vi "subItemInfoToLinkerInfo.vi"(11 "Item info[]":T1[](array[typedef])) -> (3 "Linker.Read Info From File":T3(array[cluster]))   [LabVIEW 2020, in "Tests.DependencyInspection.lvlib"]
uses:
  Tests.DependencyInspection.lvlib
  <vilib>/Utility/lvfile.llb/LVFileType.ctl
  <vilib>/Utility/lvfile.llb/NI_FileType.lvlib
  ItemInfo.ctl
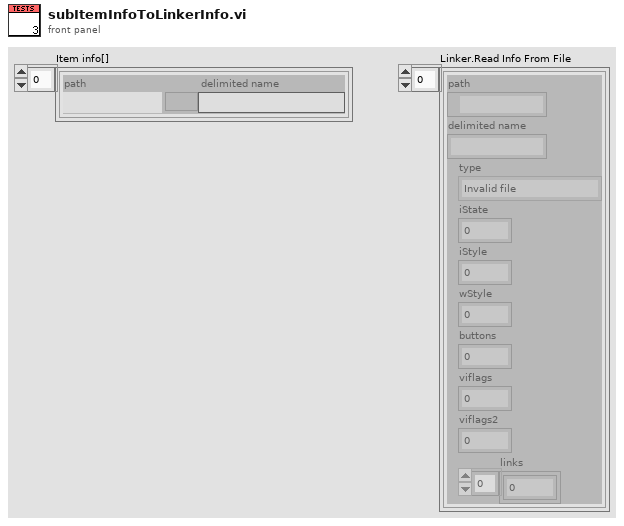
[diagram p1: front panel]
types:
  T1 = typedef "Tests.DependencyInspection.lvlib/ItemInfo.ctl" = cluster{"path":path, "delimited name":string}
  T2 = typedef "NI_FileType.lvlib/LVFileType.ctl" = enum32{"Invalid file", "Unknown type", "Instrument", "Control", "Polymorphic VI", "Project", "Library", "LVClass", "XControl", "XNode", "Shared library", ".NET assembly", "ActiveX interface", "CIN", "Run-time menu", "Palette menu", "Help file", "LLB", "XNode Edit Dependency", "Class Private Data Control", "Statechart", "MathScript .m file", "Ladder Diagram", "LVLibp", "XNode Build Dependency"}
  T3 = cluster{"path":path, "delimited name":string, "type":T2, "iState":u32, "iStyle":u16, "wStyle":u16, "buttons":u16, "viflags":u32, "viflags2":u32, "links":u32[]}[]
  T4 = cluster{"path":path, "delimited name":string, "type":T2, "iState":u32, "iStyle":u16, "wStyle":u16, "buttons":u16, "viflags":u32, "viflags2":u32, "links":u32[]}
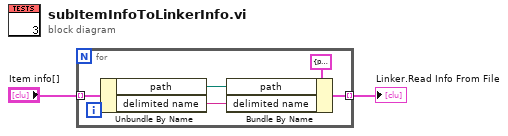
[diagram p0: block diagram]
diagram:
  n1 = for {
    tunnel: "Item info[]" -> [w5] mode=indexing
    tunnel: [w6] -> w2 mode=indexing
    n2 = Unbundle By Name(w5) -> ("path"=w4:path, "delimited name"=w3:string)
    n3 = Bundle By Name(cluster=T4 {"path"=path "", "delimited name"="", "type"=enum."Invalid file", "iState"=0, "iStyle"=0, "wStyle"=0, "buttons"=0, "viflags"=0, "viflags2"=0, "links"=[]}, "path"=w4, "delimited name"=w3) -> (w6:T4)
  }
  "Linker.Read Info From File" <- w2
